vi "PCO_ResetSettingsToDefault.vi"(8 "error in (no error)":errorcluster {"code" format="%x"}, 11 "ph":u64) -> (0 "error out":errorcluster {"code" format="%x"}, 2 "ErrorMessage":i32 format="%x", 3 "ph out":u64)   [LabVIEW 2019, in "SDK.lvlib" / "GeneralCameraControl.lvlib"]
doc: "<b>Description:</b>\nThis function can be used to reset all camera settings to its default values. This function is also executed during a power-up sequence. The camera must be stopped before calling this command. Default settings are slightly different for all cameras.\n\n<b>Supported camera type:</b>\nAll cameras\n\n<b>Descriptor dependency:</b>\nNone"
uses:
  GeneralCameraControl.lvlib
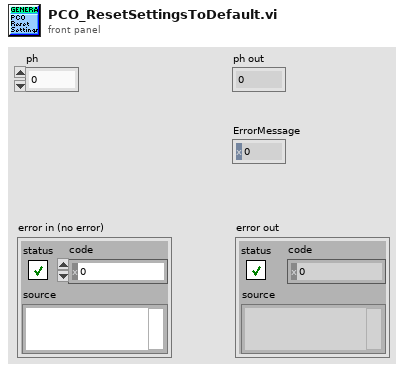
[diagram p1: front panel]
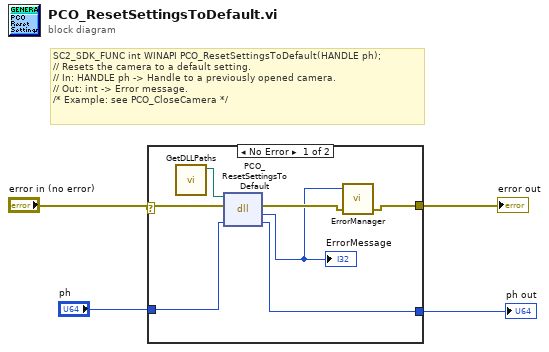
[diagram p0: block diagram]
diagram:
  # "SC2_SDK_FUNC int WINAPI PCO_ResetSettingsToDefault(HANDLE ph);\n// Resets the camera to a default setting.\n// In: HANDLE ph -> Handle to a previously opened camera.\n// Out: int -> Error message.\n/* Example: see PCO_CloseCamera */"
  n1 = case shown="No Error" "error in (no error)" {
    selector: "error in (no error)" -> [w9 w13]
    tunnel: "ph" -> [w11 w12]
    tunnel: [w10 w12] -> w3
    tunnel: [w8 w13] -> w2
    frame No Error {
      n2 = call "GetDLLPaths.vi"() -> ("SC2_Cam_Path"=w5:path)  [unwired: 9 in, 2 out]
      n3 = dll-call lib="?" fn="PCO_ResetSettingsToDefault"(path in=w5, error in=w9, "ph"=w11) -> (error out=w7:errorcluster, "return type"=w6:i32, "ph"=w10:u64)  [unwired: 1 in, 1 out]
      "ErrorMessage" <- w6
      n4 = call "ErrorManager.vi"("error in (no error)"=w7, "error code"=w6) -> ("error out"=w8:errorcluster)  [unwired: 3 in]
    }
    frame Error {
    }
  }
  "ph out" <- w3
  "error out" <- w2
